vi "write_to_text.vi"(8 "error out":errorcluster, 9 "VISA Output":refnum<visa-resource-name>, 10 "byte count":u32, 11 "refnum":refnum<file>) -> (0 "return count":u32, 1 "read buffer":string, 2 "error out 2":errorcluster, 3 "VISA resource name":refnum<visa-resource-name>)   [LabVIEW 2015]
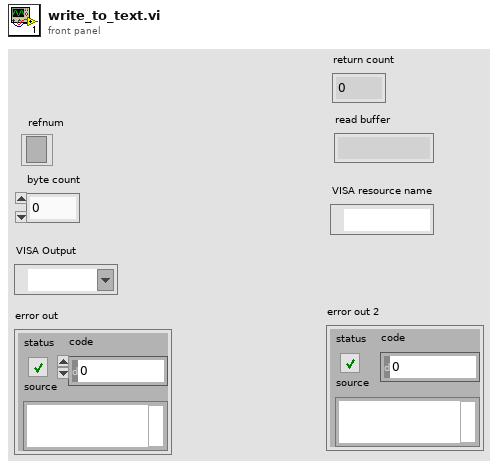
[diagram p1: front panel]
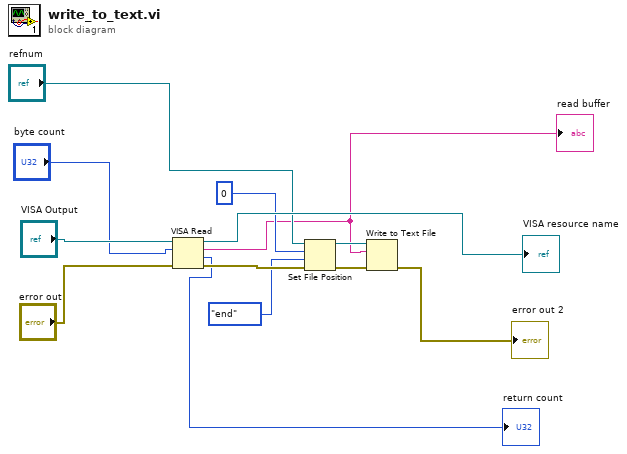
[diagram p0: block diagram]
diagram:
  n1 = VISA Read(VISA resource name="VISA Output", byte count="byte count", error in (no error)="error out") -> (VISA resource name out=→"VISA resource name":refnum<visa-resource-name>, read buffer=w2:string, return count=→"return count":u32, error out=w6:errorcluster)
  "read buffer" <- w2
  n2 = Set File Position(offset (in bytes) (0)=i64 0, refnum="refnum", from (0:start)=enum16{"start", "end", "current"}."end", error in=w6) -> (refnum out=w8:refnum<file>, error out=w7:errorcluster)
  n3 = Write to Text File(file (use dialog)=w8, text=w2, error in=w7) -> (error out=→"error out 2":errorcluster)  [unwired: 1 in, 2 out]
